vi "ScaleSquat_Depth.vi"(8 "Enum":enum16{"3D", "2D"}(ring)=enum."2D", 10 "ScalingCoef":dbl=1.0, 11 "Averaged Squat Trajectory":dbl[][](array[numeric])) -> (2 "ScaledGait":dbl[][](array[numeric]), 3 "XY Graph":cluster{"Y":dbl[], "Y":dbl[]}[](graph))   [LabVIEW 2016]
uses:
  <userlib>/_OpenG.lib/array/array.llb/Index 1D Array Elements (DBL)__ogtk.vi
  <vilib>/imath/engines/lvmath2/RunTimeEngine/IndexRead/NIMS V(S).vi
  <instcachedir>/0/NIMS V(S)_0488751826AF41519A22953C041130DC.lvgen/NIMS V(S)_0488751826AF41519A22953C041130DC_000.vi
  <vilib>/imathl/engines/lvmath/Functions/Error Handling/Create Error.vi
  <vilib>/imath/engines/lvmath2/RunTimeEngine/ArithmeticOperatorToken/NIMS_ArithmeticOperator_power(S).vi
  <instcachedir>/0/NIMS_ArithmeticOperator_power(S)_1E6AB98FD36540B9B758A69A385A1B47.lvgen/NIMS_ArithmeticOperator_power(S)_1E6AB98FD36540B9B758A69A385A1B47_015.vi
  <instcachedir>/0/NIMS_ArithmeticOperator_power(S)_1E6AB98FD36540B9B758A69A385A1B47.lvgen/NIMS_ArithmeticOperator_power(S)_1E6AB98FD36540B9B758A69A385A1B47_014.vi
  <vilib>/imath/engines/lvmath2/RunTimeEngine/ErrorHandling/NIMS_Create Error From Enums.vi
  <vilib>/imath/engines/lvmath2/RunTimeEngine/NodeEndStatement/NIMS_NodeEndStatement_Output.vi
  <instcachedir>/0/NIMS_NodeEndStatement_Output_53EC0D466D134D7ABD903AC30B43404B.lvgen/NIMS_NodeEndStatement_Output_53EC0D466D134D7ABD903AC30B43404B_005.vi
  <vilib>/imath/engines/lvmath2/RunTimeEngine/ErrorHandling/NIMS_Finalize Error.vi
panel:
  out "XY Graph 2":cluster{dbl[], "yi":dbl[]}(graph)
  out "XY":cluster{"Mean":dbl[], "Mean":dbl[]}[](array[cluster])
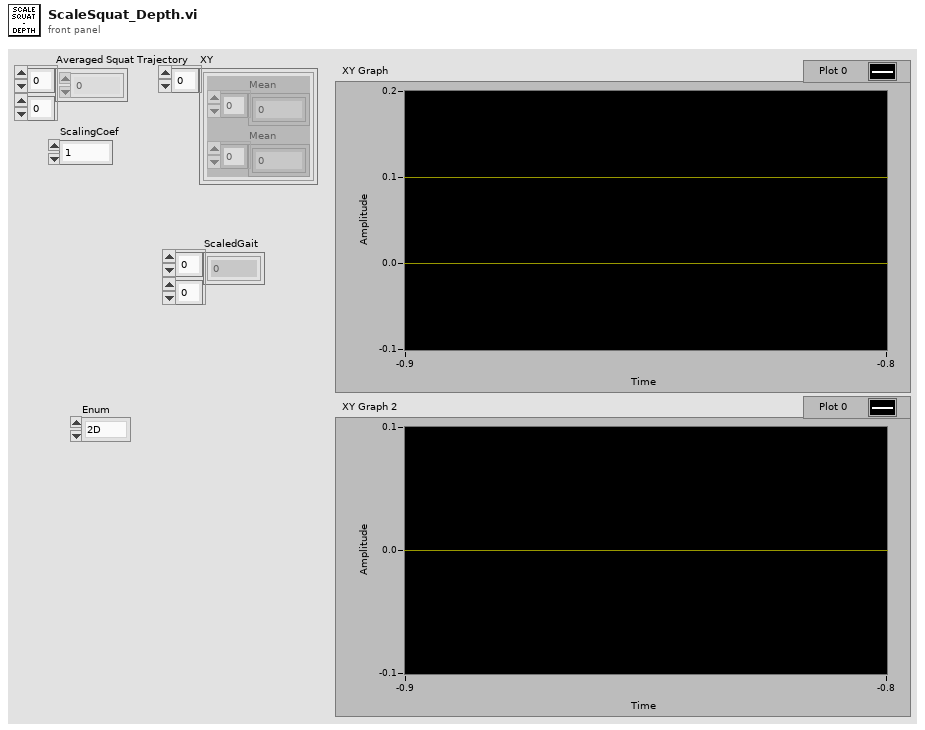
[diagram p1: front panel]
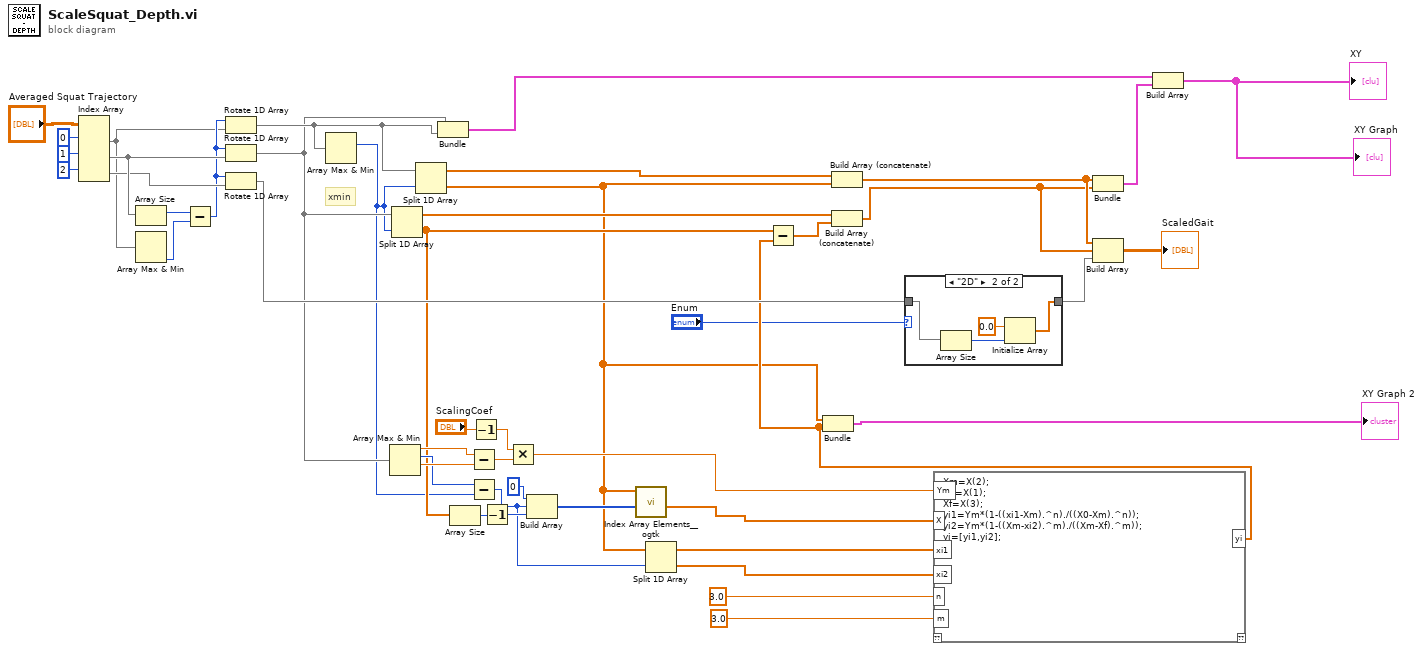
[diagram p0: block diagram]
diagram:
  # "xmin"
  n1 = Index Array(array="Averaged Squat Trajectory", index (row) #1=0 ("index (row)"), index (row) #2=1 ("index (row)"), index (row) #3=2 ("index (row)")) -> (element #1=w35:dbl[], element #2=w42:dbl[], element #3=w39:dbl[])  [unwired: 3 in]
  n2 = Array Size(array=w42) -> (size(s)=w41:i32)
  n3 = Array Max & Min(array=w35) -> (min index (indices)=w1:i32)  [unwired: 3 out]
  n4 = Subtract(x=w41, y=w1) -> (x-y=w38:i32)
  n5 = Rotate 1D Array(1:w35, 2:w38) -> (0:w6:dbl[])
  n6 = Rotate 1D Array(1:w42, 2:w38) -> (0:w5:dbl[])
  n7 = Rotate 1D Array(1:w39, 2:w38) -> (0:w36:dbl[])
  n8 = Array Max & Min(array=w6) -> (max index (indices)=w2:i32)  [unwired: 3 out]
  n9 = Array Max & Min(array=w5) -> (max value=w31:dbl, max index (indices)=w25:i32, min value=w32:dbl)  [unwired: 1 out]
  n10 = Split 1D Array(array=w5, index=w2) -> (first subarray=w29:dbl[], second subarray=w21:dbl[])
  n11 = Split 1D Array(array=w6, index=w2) -> (first subarray=w28:dbl[], second subarray=w14:dbl[])
  n12 = Bundle(w5, w6) -> (w46:cluster{dbl[], dbl[]})  [unwired: 1 in]
  n13 = Array Size(array=w21) -> (size(s)=w34:i32)
  n14 = Subtract(x=w31, y=w32) -> (x-y=w23:dbl)
  n15 = Subtract(x=w25, y=w2) -> (x-y=w13:i32)
  n16 = Decrement(x="ScalingCoef") -> (x-1=w22:dbl)
  n17 = Decrement(x=w34) -> (x-1=w24:i32)
  n18 = Multiply(x=w22, y=w23) -> (x*y=w18:dbl)
  n19 = Build Array(0 ("element"), w13, w24) -> (w19:i32[])
  n20 = call-poly <userlib>:"Index Array Elements__ogtk.vi"("indices"=w19, "array"=w14) -> ("elements"=w17:dbl[])  [unwired: 9 in]
  n21 = Split 1D Array(array=w14, index=w13) -> (first subarray=w12:dbl[], second subarray=w11:dbl[])
  n22 = Build Array (concatenate)(w28, w14) -> (w4:dbl[])
  n23 = case shown="\"2D\"" "Enum" {
    tunnel: w36 -> [w47 w51]
    tunnel: [w47 w49] -> w7
    frame "3D", Default {
    }
    frame "2D" {
      n24 = Array Size(array=w51) -> (size(s)=w50:i32)
      n25 = Initialize Array(0.0 ("element"), w50) -> (w49:dbl[])
    }
  }
  n26 = mathscript code="Xm=X(2);\nX0=X(1);\nXf=X(3);\nyi1=Ym*(1-((xi1-Xm).^n)./((X0-Xm).^n));\nyi2=Ym*(1-((Xm-xi2).^m)./((Xm-Xf).^m));\nyi=[yi1,yi2];"("Ym"=w18, "X"=w17, "xi1"=w12, "n"=3.0 ("element"), "xi2"=w11, "m"=3.0 ("element")) -> ("yi"=w15:dbl[])  [unwired: 1 in, 1 out]
  n27 = Subtract(x=w21, y=w15) -> (x-y=w30:dbl[])
  n28 = Bundle(w14, "yi"=w15) -> (→"XY Graph 2":cluster{dbl[], "yi":dbl[]})  [unwired: 1 in]
  n29 = Build Array (concatenate)(w29, w30) -> (w3:dbl[])
  n30 = Bundle(w4, w3) -> (w27:cluster{dbl[], dbl[]})  [unwired: 1 in]
  n31 = Build Array(w4, w3, w7) -> (→"ScaledGait":dbl[][])
  n32 = Build Array(w46, w27) -> (→"XY" →"XY Graph":cluster{dbl[], dbl[]}[])
